vi "start accessory panels.vi"(7 "Grabber":refnum<vi>, 8 "error in (no error)":errorcluster, 9 "stim laser ref":refnum<vi>, 10 "FPGA VI ref":T1, 11 "Queues":T3) -> (0 "error out":errorcluster, 3 "refs":T2)   [LabVIEW 2010]
uses:
  internal_queues.ctl
  line_info.ctl
  volume_with_lines.ctl
  volume_info.ctl
  kalman_result_scaled.ctl
  projection buffers.ctl
  location3D.ctl
  spot location.ctl
  FPGA_ref.ctl
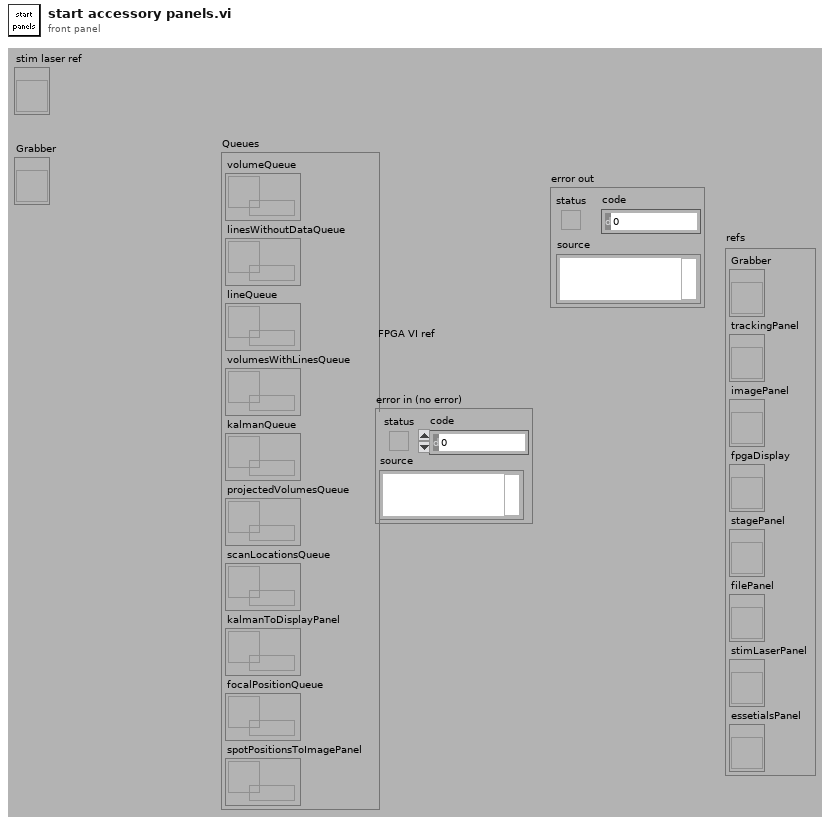
[diagram p1: front panel]
types:
  T1 = typedef "FPGA_ref.ctl" = refnum<k20>
  T2 = cluster{"Grabber":refnum<vi>, "trackingPanel":refnum<vi>, "imagePanel":refnum<vi>, "fpgaDisplay":refnum<vi>, "stagePanel":refnum<vi>, "filePanel":refnum<vi>, "stimLaserPanel":refnum<vi>, "essetialsPanel":refnum<vi>}
  T3 = typedef "internal_queues.ctl" = cluster{"volumeQueue":refnum<queue>, "linesWithoutDataQueue":refnum<queue>, "lineQueue":refnum<queue>, "volumesWithLinesQueue":refnum<queue>, "kalmanQueue":refnum<queue>, "projectedVolumesQueue":refnum<queue>, "scanLocationsQueue":refnum<queue>, "kalmanToDisplayPanel":refnum<queue>, "focalPositionQueue":refnum<queue>, "spotPositionsToImagePanel":refnum<queue>}
  T4 = cluster{"Grabber":refnum<vi>, refnum<vi>, refnum<vi>, refnum<vi>, refnum<vi>, refnum<vi>, refnum<vi>, refnum<vi>}
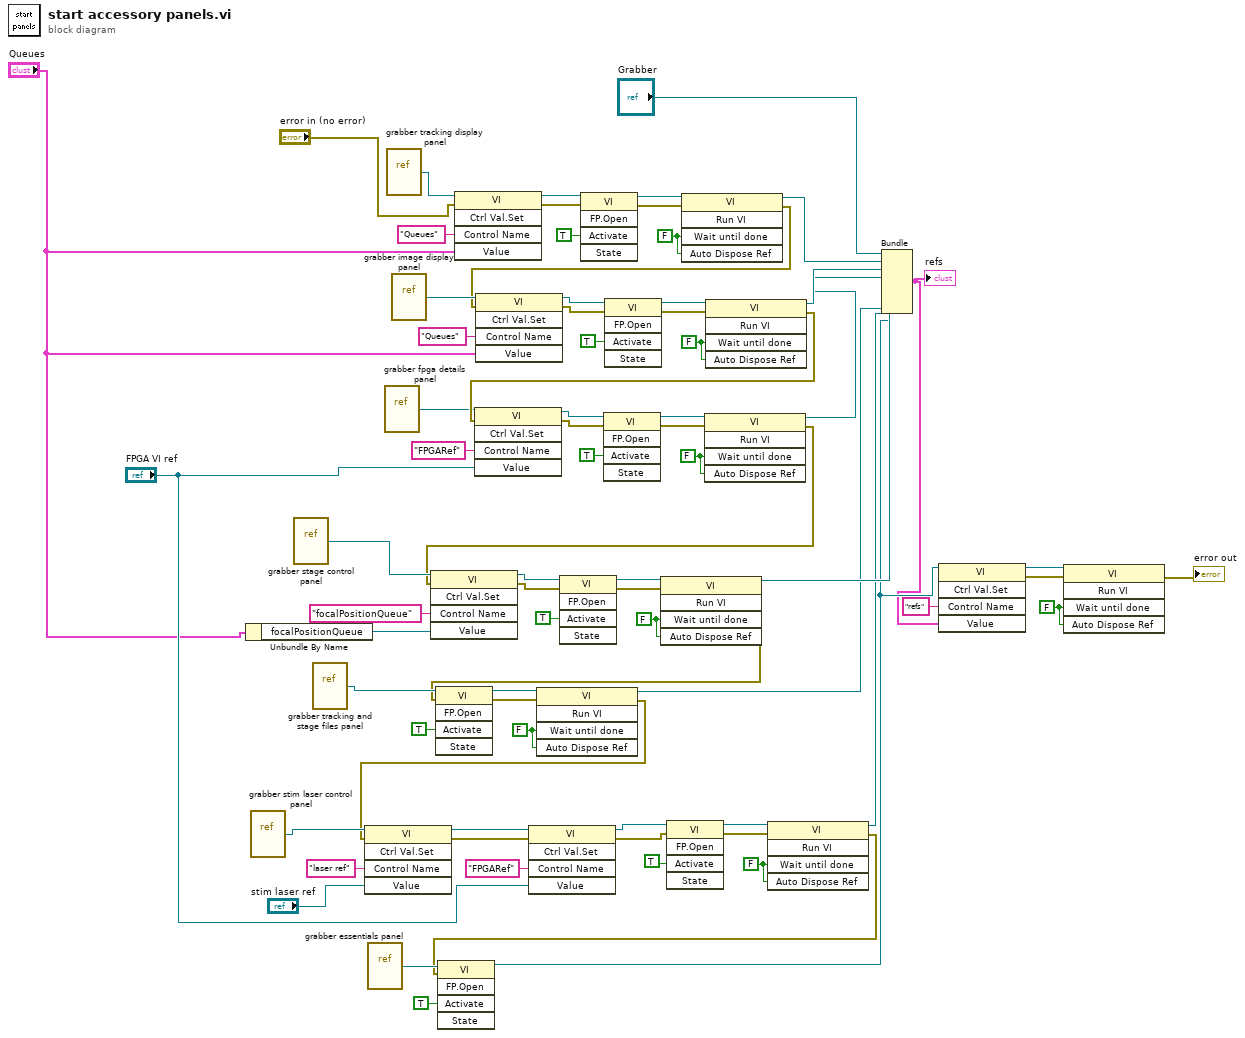
[diagram p0: block diagram]
diagram:
  w9 = FALSE ("Wait Until Done")
  w26 = FALSE ("Wait Until Done")
  w31 = FALSE ("Wait Until Done")
  w39 = FALSE ("Wait Until Done")
  w49 = FALSE ("Wait Until Done")
  w64 = FALSE ("Wait Until Done")
  w71 = FALSE ("Wait Until Done")
  n1 = Unbundle By Name("Queues") -> ("focalPositionQueue"=w36:refnum<queue>)
  n2 = vi-ref "grabber stim laser control panel.vi"() -> (w23:refnum<vi>)
  n3 = vi-ref "grabber stage control panel.vi"() -> (w38:refnum<vi>)
  n4 = vi-ref "grabber tracking and stage files panel.vi"() -> (w30:refnum<vi>)
  n5 = vi-ref "grabber essentials panel.vi"() -> (w8:refnum<vi>)
  n6 = vi-ref "grabber fpga details panel.vi"() -> (w46:refnum<vi>)
  n7 = vi-ref "grabber tracking display panel.vi"() -> (w61:refnum<vi>)
  n8 = vi-ref "grabber image display panel.vi"() -> (w59:refnum<vi>)
  n9 = invoke class="VI" method="Ctrl Val.Set"(reference=w61, error in="error in (no error)", "Control Name"="Queues", "Value"="Queues") -> (reference out=w63:refnum<vi>, error out=w62:errorcluster)  [unwired: 1 in, 3 out]
  n10 = invoke class="VI" method="FP.Open"(reference=w63, error in=w62, "Activate"=TRUE ("Activate?")) -> (reference out=w72:refnum<vi>, error out=w73:errorcluster)  [unwired: 2 in, 3 out]
  n11 = invoke class="VI" method="Run VI"(reference=w72, error in=w73, "Wait until done"=w71, "Auto Dispose Ref"=w71) -> (reference out=w57:refnum<vi>, error out=w58:errorcluster)  [unwired: 1 in, 3 out]
  n12 = invoke class="VI" method="Ctrl Val.Set"(reference=w59, error in=w58, "Control Name"="Queues", "Value"="Queues") -> (reference out=w69:refnum<vi>, error out=w68:errorcluster)  [unwired: 1 in, 3 out]
  n13 = invoke class="VI" method="FP.Open"(reference=w69, error in=w68, "Activate"=TRUE ("Activate?")) -> (reference out=w65:refnum<vi>, error out=w66:errorcluster)  [unwired: 2 in, 3 out]
  n14 = invoke class="VI" method="Run VI"(reference=w65, error in=w66, "Wait until done"=w64, "Auto Dispose Ref"=w64) -> (reference out=w56:refnum<vi>, error out=w48:errorcluster)  [unwired: 1 in, 3 out]
  n15 = invoke class="VI" method="Ctrl Val.Set"(reference=w46, error in=w48, "Control Name"="FPGARef", "Value"="FPGA VI ref") -> (reference out=w54:refnum<vi>, error out=w53:errorcluster)  [unwired: 1 in, 3 out]
  n16 = invoke class="VI" method="FP.Open"(reference=w54, error in=w53, "Activate"=TRUE ("Activate?")) -> (reference out=w50:refnum<vi>, error out=w51:errorcluster)  [unwired: 2 in, 3 out]
  n17 = invoke class="VI" method="Run VI"(reference=w50, error in=w51, "Wait until done"=w49, "Auto Dispose Ref"=w49) -> (reference out=w47:refnum<vi>, error out=w37:errorcluster)  [unwired: 1 in, 3 out]
  n18 = invoke class="VI" method="Ctrl Val.Set"(reference=w38, error in=w37, "Control Name"="focalPositionQueue", "Value"=w36) -> (reference out=w44:refnum<vi>, error out=w43:errorcluster)  [unwired: 1 in, 3 out]
  n19 = invoke class="VI" method="FP.Open"(reference=w44, error in=w43, "Activate"=TRUE ("Activate?")) -> (reference out=w40:refnum<vi>, error out=w41:errorcluster)  [unwired: 2 in, 3 out]
  n20 = invoke class="VI" method="Run VI"(reference=w40, error in=w41, "Wait until done"=w39, "Auto Dispose Ref"=w39) -> (reference out=w35:refnum<vi>, error out=w29:errorcluster)  [unwired: 1 in, 3 out]
  n21 = invoke class="VI" method="FP.Open"(reference=w30, error in=w29, "Activate"=TRUE ("Activate?")) -> (reference out=w32:refnum<vi>, error out=w33:errorcluster)  [unwired: 2 in, 3 out]
  n22 = invoke class="VI" method="Run VI"(reference=w32, error in=w33, "Wait until done"=w31, "Auto Dispose Ref"=w31) -> (reference out=w28:refnum<vi>, error out=w20:errorcluster)  [unwired: 1 in, 3 out]
  n23 = invoke class="VI" method="Ctrl Val.Set"(reference=w23, error in=w20, "Control Name"="laser ref", "Value"="stim laser ref") -> (reference out=w17:refnum<vi>, error out=w14:errorcluster)  [unwired: 1 in, 3 out]
  n24 = invoke class="VI" method="Ctrl Val.Set"(reference=w17, error in=w14, "Control Name"="FPGARef", "Value"="FPGA VI ref") -> (reference out=w16:refnum<vi>, error out=w15:errorcluster)  [unwired: 1 in, 3 out]
  n25 = invoke class="VI" method="FP.Open"(reference=w16, error in=w15, "Activate"=TRUE ("Activate?")) -> (reference out=w24:refnum<vi>, error out=w25:errorcluster)  [unwired: 2 in, 3 out]
  n26 = invoke class="VI" method="Run VI"(reference=w24, error in=w25, "Wait until done"=w26, "Auto Dispose Ref"=w26) -> (reference out=w19:refnum<vi>, error out=w7:errorcluster)  [unwired: 1 in, 3 out]
  n27 = invoke class="VI" method="FP.Open"(reference=w8, error in=w7, "Activate"=TRUE ("Activate?")) -> (reference out=w3:refnum<vi>)  [unwired: 2 in, 4 out]
  n28 = Bundle("Grabber"="Grabber", w57, w56, w47, w35, w28, w19, w3) -> (w1:T4)  [unwired: 1 in]
  "refs" <- w1
  n29 = invoke class="VI" method="Ctrl Val.Set"(reference=w3, "Control Name"="refs", "Value"=w1) -> (reference out=w4:refnum<vi>, error out=w5:errorcluster)  [unwired: 2 in, 3 out]
  n30 = invoke class="VI" method="Run VI"(reference=w4, error in=w5, "Wait until done"=w9, "Auto Dispose Ref"=w9) -> (error out=→"error out":errorcluster)  [unwired: 1 in, 4 out]
